vi "main.vi"() -> ()   [LabVIEW 2020, in "Coarse Approach.lvclass"]
uses:
  Coarse Approach.lvclass
  Coarse Approach.lvclass/Coarse Approach.ctl
  Picomotor/Picomotor.lvclass
panel:
  in  "Position (steps)":dbl
  in  "fine_approach\nsetpoint":dbl=0.9
  in  "Fine Approach":bool
  in  "Quick Approach":bool
  in  "quick_approach\nsetpoint":dbl=0.99
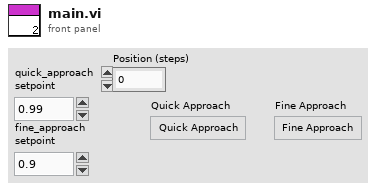
[diagram p1: front panel]
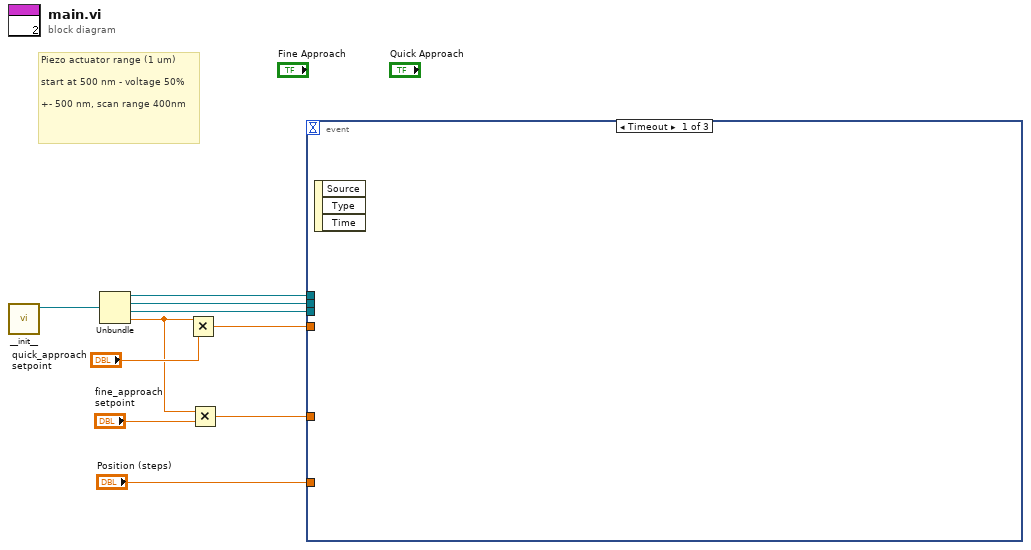
[diagram p0: block diagram]
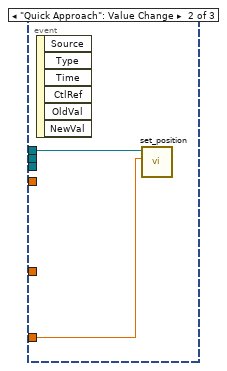
[diagram p2: hidden frame]
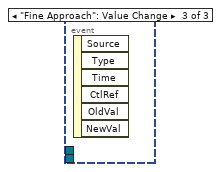
[diagram p3: hidden frame]
diagram:
  # "Piezo actuator range (1 um)\n\nstart at 500 nm - voltage 50%\n\n+- 500 nm, scan range 400nm"
  n1 = call "__init__.vi"() -> ("Coarse Approach.lvclass"=w10:refnum<class "Coarse Approach.lvclass">)  [unwired: 10 in, 1 out]
  n2 = Unbundle(w10) -> (w4:refnum<class "Picomotor.lvclass">, w3:refnum<class "Lock-In Amplifier.lvclass">, w2:refnum<class "PZT.lvclass">, w7:dbl)
  n3 = Multiply(x=w7, y="quick_approach\nsetpoint") -> (x*y=w5:dbl)
  n4 = Multiply(x=w7, y="fine_approach\nsetpoint") -> (x*y=w6:dbl)
  n5 = event shown="[0] Timeout" {
    selector: _ -> [_ _ _]
    dyn-events: _ -> [_ _ _]
    timeout: _ -> [_ _ _]
    tunnel: w6 -> [_ _ _]
    tunnel: w5 -> [_ _ _]
    tunnel: w4 -> [_ w12 _]
    tunnel: w3 -> [_ _ _]
    tunnel: w2 -> [_ _ _]
    tunnel: "Position (steps)" -> [_ w11 _]
    event Timeout {
      n6 = event-data() -> ()  [unwired: 1 in, 3 out]
    }
    event "Quick Approach": Value Change {
      n7 = event-data() -> ()  [unwired: 1 in, 6 out]
      n8 = call "set_position.vi"("Position (steps)"=w11, "Picomotor in"=w12) -> ()  [unwired: 8 in, 2 out]
    }
    event "Fine Approach": Value Change {
      n9 = event-data() -> ()  [unwired: 1 in, 6 out]
    }
  }
